vi "breakWaveform.vi"(6 "ChannelNumber":i32, 8 "error in (no error)":errorcluster, 9 "samplingRate":dbl, 10 "total duration":dbl, 11 "SoundDeviceData in":refnum<class "SoundDeviceData.lvclass">) -> (0 "error out":errorcluster, 1 "samplePerChunkPerChannel":dbl, 2 "samplesPerChannelTotal":dbl, 3 "SoundDeviceData out":refnum<class "SoundDeviceData.lvclass">)   [LabVIEW 2011, in "DataMappers.lvlib" / "SoundDeviceData.lvclass"]
uses:
  SoundDeviceData.lvclass
  SoundDeviceData.lvclass/SoundDeviceData.ctl
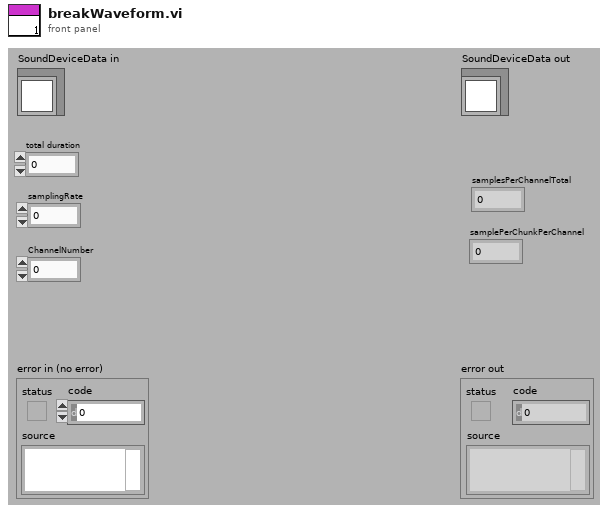
[diagram p1: front panel]
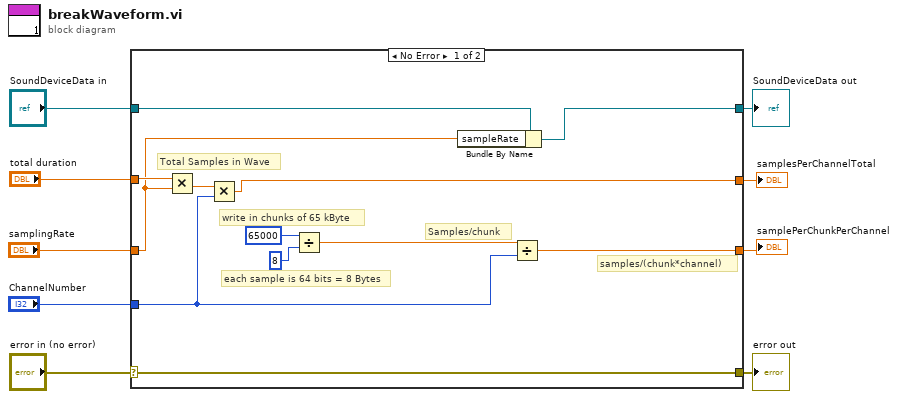
[diagram p0: block diagram]
diagram:
  n1 = case shown="No Error" "error in (no error)" {
    selector: "error in (no error)" -> [w21 w23]
    tunnel: [w21 w23] -> w8
    tunnel: [w10 w22] -> w6
    tunnel: "SoundDeviceData in" -> [w11 w22]
    tunnel: "total duration" -> [w20 _]
    tunnel: "samplingRate" -> [w12 _]
    tunnel: "ChannelNumber" -> [w14 _]
    tunnel: [w13 _] -> w2
    tunnel: [w16 _] -> w1
    frame No Error {
      # "samples/(chunk*channel)"
      # "Samples/chunk"
      # "each sample is 64 bits = 8 Bytes"
      # "write in chunks of 65 kByte"
      # "Total Samples in Wave"
      n2 = Multiply(x=w20, y=w12) -> (x*y=w19:dbl)
      n3 = Multiply(x=w19, y=w14) -> (x*y=w16:dbl)
      n4 = Divide(x=65000, y=8) -> (x/y=w15:dbl)
      n5 = Bundle By Name(cluster=w11, "sampleRate"=w12) -> (w10:refnum<class "SoundDeviceData.lvclass">)
      n6 = Divide(x=w15, y=w14) -> (x/y=w13:dbl)
    }
    frame Error {
    }
  }
  "error out" <- w8
  "SoundDeviceData out" <- w6
  "samplesPerChannelTotal" <- w1
  "samplePerChunkPerChannel" <- w2
